vi "Curseur_Position.vi"(8 "error in (no error)":errorcluster caption="entrée d'erreur (pas d'erreur)", 11 "Data Cam Processing":T2 {"sigma X" format="%0.2f"; "mean X" format="%0.2f"; "mean Y" format="%0.2f"; "sigma Y" format="%0.2f"; "Shutter (us)" scale=22.0..10000000.0; "Gain Caméra" scale=0.0..1023.0}) -> (0 "error out":errorcluster caption="sortie d'erreur", 2 "Curseur":T1, 3 "Data Cam Processing 2":T2 {"sigma X" format="%0.2f"; "mean X" format="%0.2f"; "mean Y" format="%0.2f"; "sigma Y" format="%0.2f"; "Shutter (us)" scale=22.0..10000000.0; "Gain Caméra" scale=0.0..1023.0})   [LabVIEW 2026]
uses:
  Data-Processing.ctl
  <vilib>/Serenial/G Industrial Camera/g_industrial_cam/Buffer/Buffer.lvclass
  <vilib>/Serenial/G Industrial Camera/g_industrial_cam/Camera/Camera.lvclass
  <vilib>/picture/picture.llb/imagedata.ctl
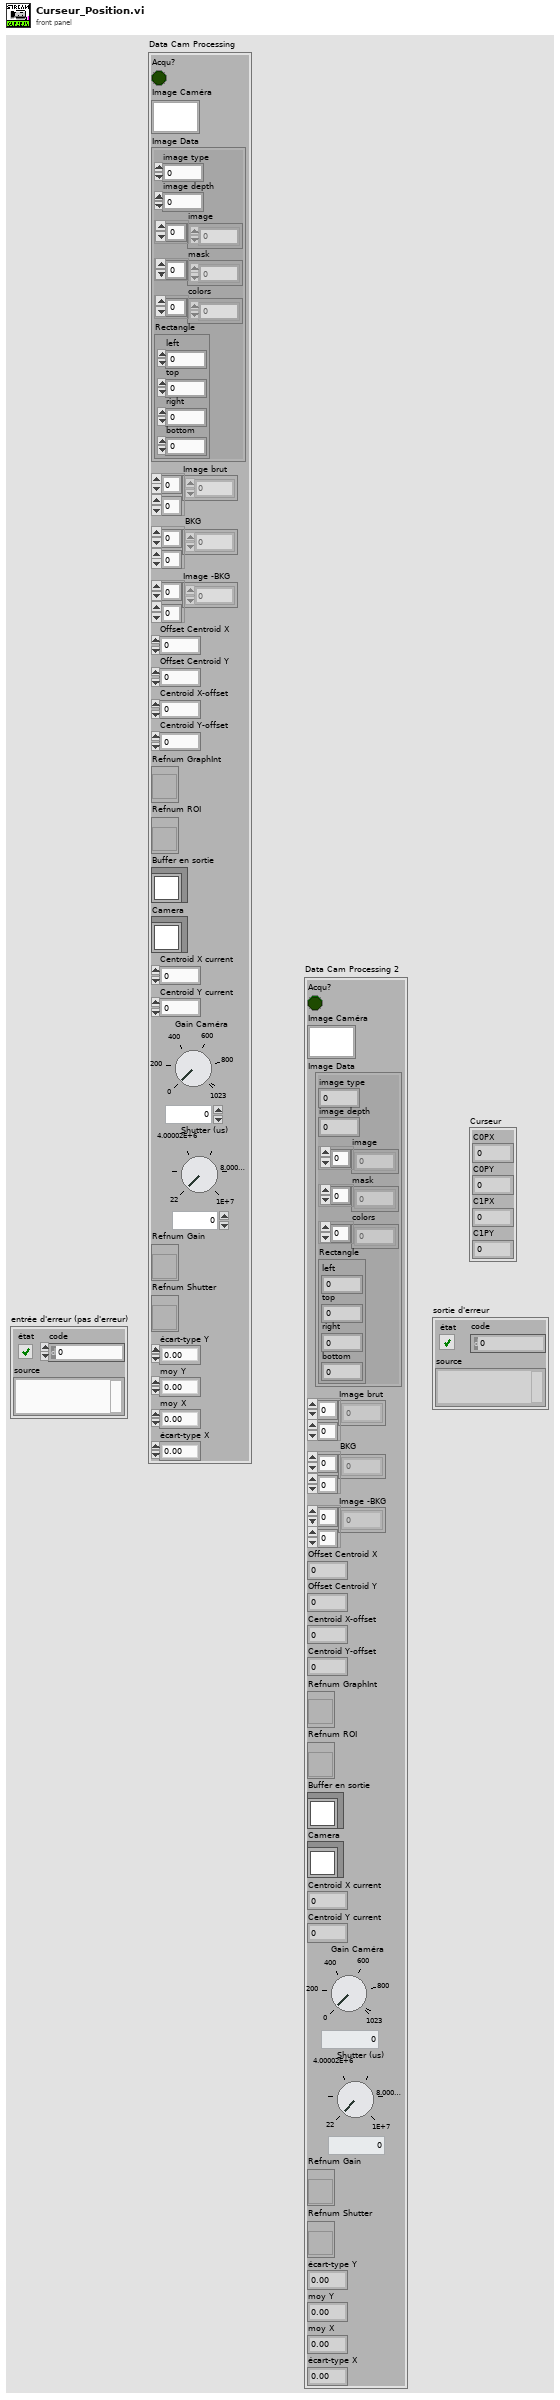
[diagram p1: front panel]
types:
  T1 = cluster{"C0PX":dbl, "C0PY":dbl, "C1PX":dbl, "C1PY":dbl}
  T2 = typedef "Data-Processing.ctl" = cluster{"Acqu?":bool, "Image Caméra":picture, "Image Data":T3, "Image brut":i16[][], "BKG":i16[][], "Image -BKG":i16[][], "Offset Centroid X":dbl, "Offset Centroid Y":dbl, "Centroid X-offset":dbl, "Centroid Y-offset":dbl, "Refnum GraphInt":refnum<vi>, "Refnum ROI":refnum<vi>, "Buffer en sortie":refnum<class "Buffer.lvclass">, "Camera":refnum<class "Camera.lvclass">, "Centroid X current":dbl, "Centroid Y current":dbl, "Gain Caméra":i32, "Shutter (us)":dbl, "Refnum Gain":refnum<vi>, "Refnum Shutter":refnum<vi>, "sigma Y":dbl, "mean Y":dbl, "mean X":dbl, "sigma X":dbl}
  T3 = typedef "imagedata.ctl" = cluster{"image type":i32, "image depth":i32, "image":u8[], "mask":u8[], "colors":u32[], "Rectangle":cluster{"left":i16, "top":i16, "right":i16, "bottom":i16}}
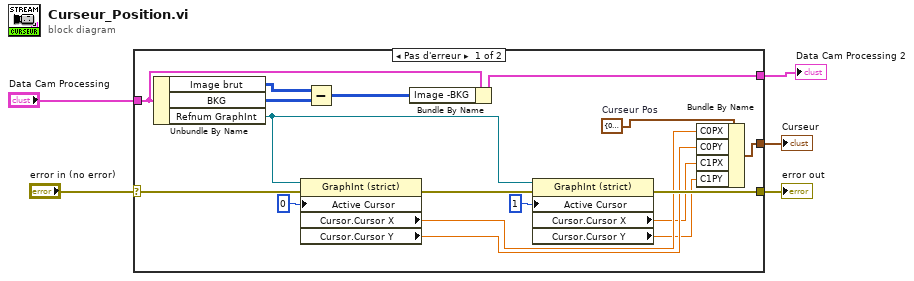
[diagram p0: block diagram]
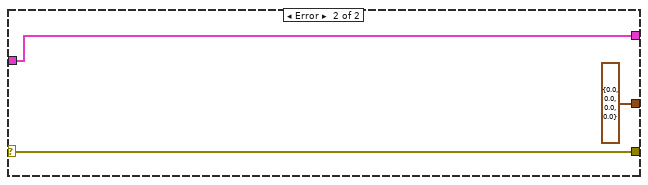
[diagram p2: hidden frame]
diagram:
  n1 = case shown="Pas d'erreur" "error in (no error)" {
    selector: "error in (no error)" -> [w21 w25]
    tunnel: [w19 w25] -> w4
    tunnel: [w14 w24] -> w3
    tunnel: "Data Cam Processing" -> [w15 w24]
    tunnel: [w8 T1 {"C0PX"=0.0, "C0PY"=0.0, "C1PX"=0.0, "C1PY"=0.0} ("Curseur Pos")] -> w1
    frame No Error {
      w13 = T1 {"C0PX"=0.0, "C0PY"=0.0, "C1PX"=0.0, "C1PY"=0.0}  # Curseur Pos
      n2 = Unbundle By Name(w15) -> ("Image brut"=w7:i16[][], "BKG"=w6:i16[][], "Refnum GraphInt"=w18:refnum<vi>)
      n3 = property class="GraphInt (strict)"(reference=w18, error in=w21, "Active Cursor"=u32 0 ("Curseur actif")) -> (error out=w20:errorcluster, "Cursor.Cursor X"=w12:dbl, "Cursor.Cursor Y"=w11:dbl)  [unwired: 1 out]
      n4 = Subtract(x=w7, y=w6) -> (x-y=w16:i16[][])
      n5 = Bundle By Name(cluster=w15, "Image -BKG"=w16) -> (w14:T2)
      n6 = property class="GraphInt (strict)"(reference=w18, error in=w20, "Active Cursor"=u32 1 ("Curseur actif")) -> (error out=w19:errorcluster, "Cursor.Cursor X"=w10:dbl, "Cursor.Cursor Y"=w9:dbl)  [unwired: 1 out]
      n7 = Bundle By Name(cluster=w13, "C0PX"=w12, "C0PY"=w11, "C1PX"=w10, "C1PY"=w9) -> (w8:T1)
    }
    frame Error {
    }
  }
  "error out" <- w4
  "Data Cam Processing 2" <- w3
  "Curseur" <- w1
